vi "Read.vi"(7 "Ignore Control":T1={"Ignore Conn Closed"=TRUE, "Ignore Timeout"=TRUE, "Ignore Corrupt Data"=TRUE}, 8 "error in (no error)":errorcluster, 10 "max size (548)":i32=548, 11 "UDP Base in":T2) -> (0 "error out":errorcluster, 1 "Network Location":T4, 2 "Receive Data":string, 3 "UDP Base out":T2, 4 "Timeout":bool, 6 "Error Code Out":i32)   [LabVIEW 2011]
uses:
  UDP Network Location.ctl
  UDP Base.ctl
  UDP Socket Params.ctl
  Ignore Control Cluster.ctl
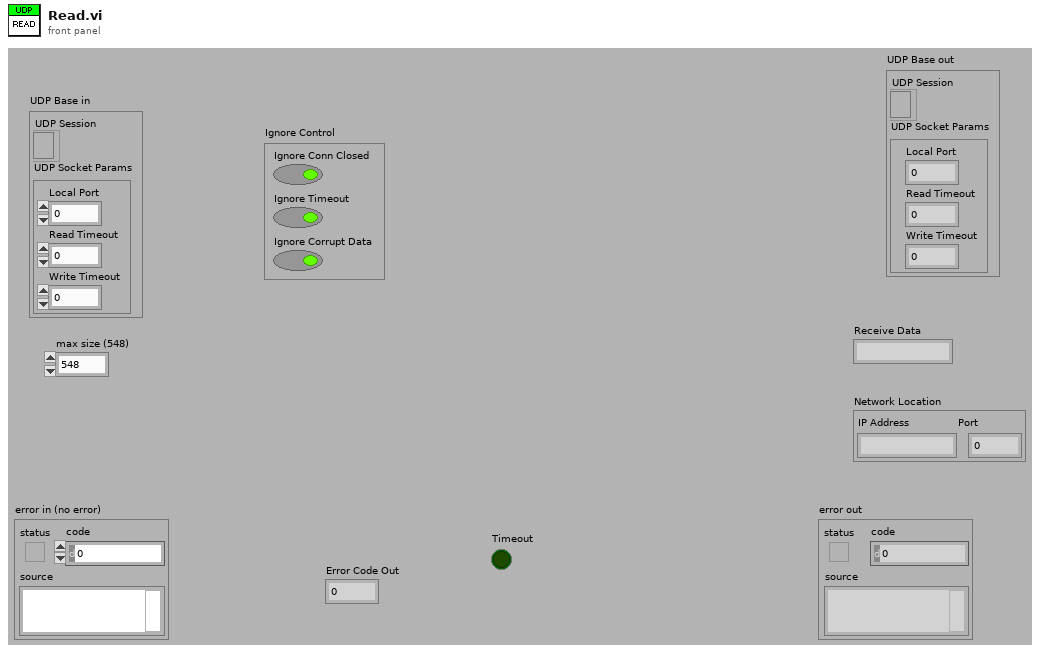
[diagram p1: front panel]
types:
  T1 = typedef "Ignore Control Cluster.ctl" = cluster{"Ignore Conn Closed":bool, "Ignore Timeout":bool, "Ignore Corrupt Data":bool}
  T2 = typedef "UDP Base.ctl" = cluster{"UDP Session":refnum<k16>, "UDP Socket Params":T3}
  T3 = typedef "UDP Socket Params.ctl" = cluster{"Local Port":u16, "Read Timeout":i32, "Write Timeout":i32}
  T4 = typedef "UDP Network Location.ctl" = cluster{"IP Address":string, "Port":u16}
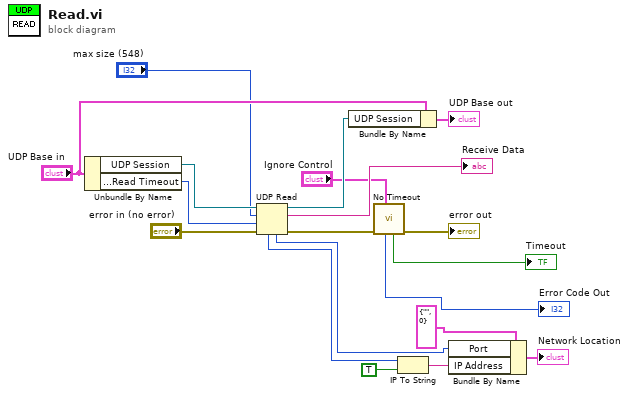
[diagram p0: block diagram]
diagram:
  n1 = Unbundle By Name("UDP Base in") -> ("UDP Session"=w19:refnum<k16>, "UDP Socket Params.Read Timeout"=w18:i32)
  n2 = UDP Read(connection ID=w19, max size (548)="max size (548)", timeout ms (25000)=w18, 8:"error in (no error)") -> (data out=→"Receive Data":string, error out=w16:errorcluster, 3:w7:refnum<k16>, 4:w9:u16, 6:w12:u32)
  n3 = Bundle By Name(cluster="UDP Base in", "UDP Session"=w7) -> (→"UDP Base out":T2)
  n4 = call "No Timeout.vi"("Ignore Control"="Ignore Control", "error in (no error)"=w16) -> ("error out"=→"error out":errorcluster, "Timeout"=→"Timeout":bool, "Error Code Out"=→"Error Code Out":i32)  [unwired: 1 in, 6 out]
  n5 = IP To String(1:TRUE ("dot notation? (F)"), 2:w12) -> (0:w11:string)
  n6 = Bundle By Name(cluster=T4 {"IP Address"="", "Port"=0} ("Network Location"), "Port"=w9, "IP Address"=w11) -> (→"Network Location":T4)
